vi "Initialize.vi"(8 "error in":errorcluster, 9 "Number of Channels":u32=1, 10 "Plugin Name":string, 11 "Cycler in":refnum<class "Cycler.lvclass">) -> (0 "error out":errorcluster, 3 "Cycler out":refnum<class "Cycler.lvclass">)   [LabVIEW 2023, in "Cycler.lvclass"]
doc: "This VI initializes required data channels for a Cycler. Wire the number of power output channels to <b>Number of Channels</b>, the default is 1."
uses:
  Cycler.lvclass
  Cycler.lvclass/Cycler.ctl
  <vilib>/ADAS Replay HIL/Channels/Tag Wrapper/Polymorphic/Open Producer Tag (Double).vi
  <vilib>/ADAS Replay HIL/Channels/Tag Wrapper/Polymorphic/Set Default Value (Double).vi
  <vilib>/ADAS Replay HIL/Channels/Tag Wrapper/Polymorphic/Open Consumer Tag (Boolean).vi
  <vilib>/ADAS Replay HIL/Channels/Tag Wrapper/Polymorphic/Set Default Value (Boolean).vi
  <vilib>/ADAS Replay HIL/Channels/Tag Wrapper/Polymorphic/Open Producer Tag (Boolean).vi
  <vilib>/ADAS Replay HIL/Channels/Tag Wrapper/Polymorphic/Open Producer Tag (Double).vi/45cd6eaa-a1ce-41a4-8aba-62a49d103d7e.vi
  <vilib>/ADAS Replay HIL/Channels/Tag Wrapper/Polymorphic/Set Default Value (Double).vi/228e99de-6fcf-414d-86fc-dc277c7b351f.vi
  <vilib>/ADAS Replay HIL/Channels/Tag Wrapper/Polymorphic/Open Consumer Tag (Boolean).vi/bacb721e-673a-491a-accd-959f2e1f334e.vi
  <vilib>/ADAS Replay HIL/Channels/Tag Wrapper/Polymorphic/Set Default Value (Boolean).vi/228e99de-6fcf-414d-86fc-dc277c7b351f.vi
  <vilib>/ADAS Replay HIL/Channels/Tag Wrapper/Polymorphic/Open Producer Tag (Boolean).vi/45cd6eaa-a1ce-41a4-8aba-62a49d103d7e.vi
  <vilib>/ADAS Replay HIL/Channels/Tag Wrapper/Polymorphic/Open Producer Tag (Double).vi/45cd6eaa-a1ce-41a4-8aba-62a49d103d7e.vi/c28b0ead-42ad-4072-80a2-aca7f2bd7ce3.vi
  <vilib>/ADAS Replay HIL/Channels/Tag Wrapper/Polymorphic/Set Default Value (Double).vi/228e99de-6fcf-414d-86fc-dc277c7b351f.vi/4bc1c15b-36ab-481f-b8dd-c64075ce723a.vi
  <vilib>/ADAS Replay HIL/Channels/Tag Wrapper/Polymorphic/Open Consumer Tag (Boolean).vi/bacb721e-673a-491a-accd-959f2e1f334e.vi/c28b0ead-42ad-4072-80a2-aca7f2bd7ce3.vi
  <vilib>/ADAS Replay HIL/Channels/Tag Wrapper/Polymorphic/Set Default Value (Boolean).vi/228e99de-6fcf-414d-86fc-dc277c7b351f.vi/4bc1c15b-36ab-481f-b8dd-c64075ce723a.vi
  <vilib>/ADAS Replay HIL/Channels/Tag Wrapper/Polymorphic/Open Producer Tag (Boolean).vi/45cd6eaa-a1ce-41a4-8aba-62a49d103d7e.vi/c28b0ead-42ad-4072-80a2-aca7f2bd7ce3.vi
  <vilib>/ADAS Replay HIL/AdasHilServices/AdasHilServices Fill In Error Info Ex.vi
  <vilib>/ADAS Replay HIL/Channels/Tag Wrapper/Tag Wrapper.lvlib
  Utilities/Utilities.lvlib
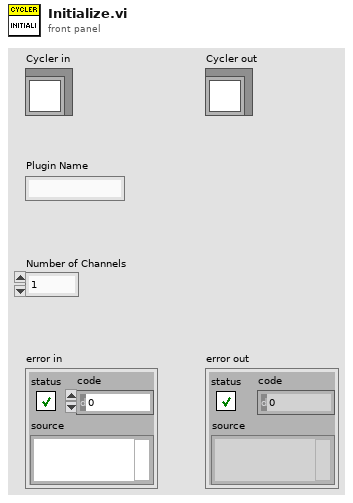
[diagram p1: front panel]
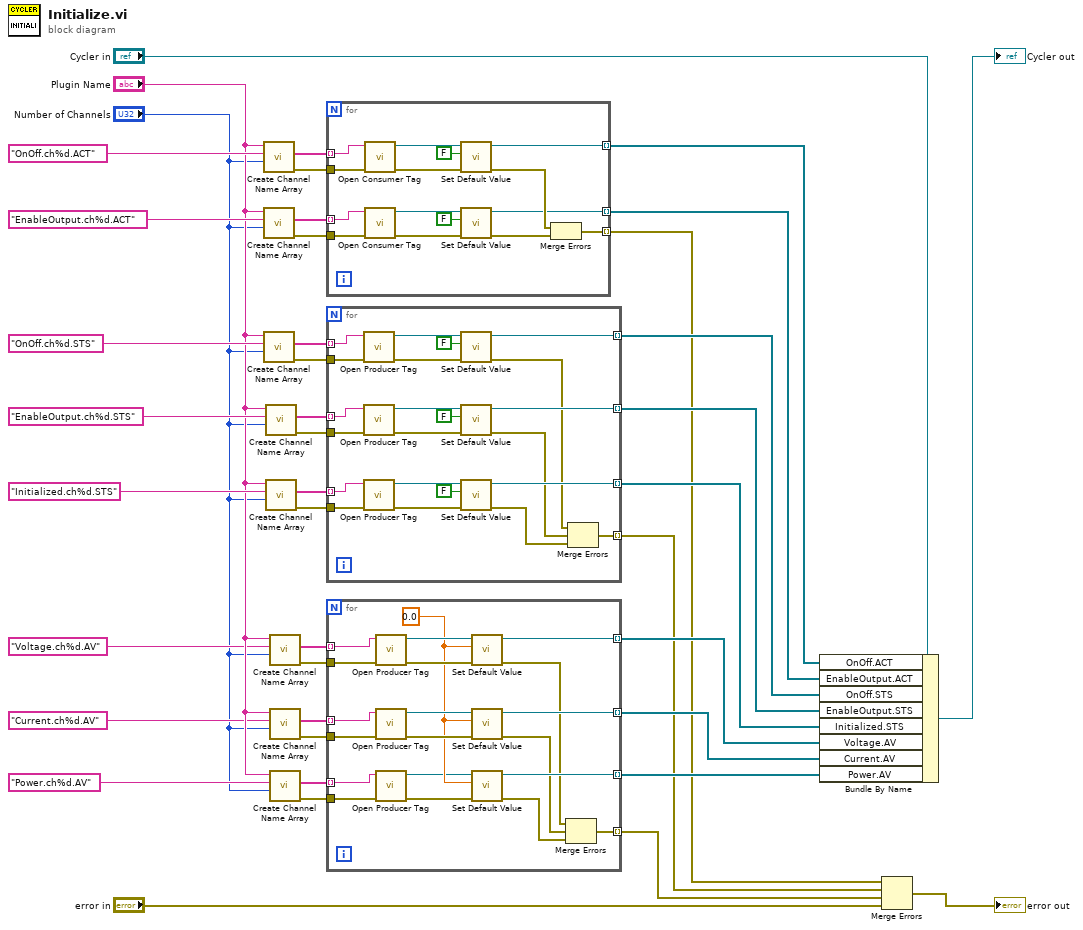
[diagram p0: block diagram]
diagram:
  n1 = call "Create Channel Name Array.vi"("Number of Channels"="Number of Channels", "Channel Format String"="OnOff.ch%d.ACT", "Plugin Name"="Plugin Name") -> ("error out"=w37:errorcluster, "Channel Names"=w40:string[])  [unwired: 7 in]
  n2 = call "Create Channel Name Array.vi"("Number of Channels"="Number of Channels", "Channel Format String"="EnableOutput.ch%d.ACT", "Plugin Name"="Plugin Name") -> ("error out"=w35:errorcluster, "Channel Names"=w34:string[])  [unwired: 7 in]
  n3 = call "Create Channel Name Array.vi"("Number of Channels"="Number of Channels", "Channel Format String"="OnOff.ch%d.STS", "Plugin Name"="Plugin Name") -> ("error out"=w32:errorcluster, "Channel Names"=w33:string[])  [unwired: 7 in]
  n4 = call "Create Channel Name Array.vi"("Number of Channels"="Number of Channels", "Channel Format String"="EnableOutput.ch%d.STS", "Plugin Name"="Plugin Name") -> ("error out"=w36:errorcluster, "Channel Names"=w39:string[])  [unwired: 7 in]
  n5 = call "Create Channel Name Array.vi"("Number of Channels"="Number of Channels", "Channel Format String"="Initialized.ch%d.STS", "Plugin Name"="Plugin Name") -> ("error out"=w27:errorcluster, "Channel Names"=w25:string[])  [unwired: 7 in]
  n6 = call "Create Channel Name Array.vi"("Number of Channels"="Number of Channels", "Channel Format String"="Voltage.ch%d.AV", "Plugin Name"="Plugin Name") -> ("error out"=w17:errorcluster, "Channel Names"=w18:string[])  [unwired: 7 in]
  n7 = call "Create Channel Name Array.vi"("Number of Channels"="Number of Channels", "Channel Format String"="Current.ch%d.AV", "Plugin Name"="Plugin Name") -> ("error out"=w15:errorcluster, "Channel Names"=w16:string[])  [unwired: 7 in]
  n8 = call "Create Channel Name Array.vi"("Number of Channels"="Number of Channels", "Channel Format String"="Power.ch%d.AV", "Plugin Name"="Plugin Name") -> ("error out"=w13:errorcluster, "Channel Names"=w14:string[])  [unwired: 7 in]
  n9 = for {
    tunnel: w40 -> [w56] mode=indexing
    tunnel: w37 -> [w55]
    tunnel: w35 -> [w54]
    tunnel: w34 -> [w53] mode=indexing
    tunnel: [w44] -> w6 mode=indexing
    tunnel: [w43] -> w5 mode=indexing
    tunnel: [w42] -> w4 mode=indexing
    n10 = call-poly <vilib>:"Open Consumer Tag.vi"("error in"=w55, "Channel Name"=w56) -> ("error out"=w51:errorcluster, "ADAS HIL Channel"=w52:refnum<k21>)  [unwired: 8 in]
    n11 = call-poly <vilib>:"Open Consumer Tag.vi"("error in"=w54, "Channel Name"=w53) -> ("error out"=w49:errorcluster, "ADAS HIL Channel"=w50:refnum<k21>)  [unwired: 8 in]
    n12 = call-poly <vilib>:"Set Default Value.vi"("error in"=w51, "Default Value"=FALSE, "ADAS HIL Channel in"=w52) -> ("error out"=w46:errorcluster, "ADAS HIL Channel out"=w43:refnum<k21>)  [unwired: 7 in]
    n13 = call-poly <vilib>:"Set Default Value.vi"("error in"=w49, "Default Value"=FALSE, "ADAS HIL Channel in"=w50) -> ("error out"=w45:errorcluster, "ADAS HIL Channel out"=w44:refnum<k21>)  [unwired: 7 in]
    n14 = Merge Errors(w46, w45) -> (w42:errorcluster)
  }
  n15 = for {
    tunnel: w39 -> [w78] mode=indexing
    tunnel: w36 -> [w77]
    tunnel: w33 -> [w76] mode=indexing
    tunnel: w32 -> [w75]
    tunnel: w27 -> [w74]
    tunnel: w25 -> [w73] mode=indexing
    tunnel: [w63] -> w7 mode=indexing
    tunnel: [w62] -> w8 mode=indexing
    tunnel: [w61] -> w9 mode=indexing
    tunnel: [w57] -> w3 mode=indexing
    n16 = call-poly <vilib>:"Open Producer Tag.vi"("error in"=w75, "Channel Name"=w76) -> ("error out"=w67:errorcluster, "ADAS HIL Channel"=w68:refnum<k21>)  [unwired: 8 in]
    n17 = call-poly <vilib>:"Open Producer Tag.vi"("error in"=w77, "Channel Name"=w78) -> ("error out"=w70:errorcluster, "ADAS HIL Channel"=w69:refnum<k21>)  [unwired: 8 in]
    n18 = call-poly <vilib>:"Open Producer Tag.vi"("error in"=w74, "Channel Name"=w73) -> ("error out"=w72:errorcluster, "ADAS HIL Channel"=w71:refnum<k21>)  [unwired: 8 in]
    n19 = call-poly <vilib>:"Set Default Value.vi"("error in"=w67, "Default Value"=FALSE, "ADAS HIL Channel in"=w68) -> ("error out"=w60:errorcluster, "ADAS HIL Channel out"=w63:refnum<k21>)  [unwired: 7 in]
    n20 = call-poly <vilib>:"Set Default Value.vi"("error in"=w70, "Default Value"=FALSE, "ADAS HIL Channel in"=w69) -> ("error out"=w59:errorcluster, "ADAS HIL Channel out"=w62:refnum<k21>)  [unwired: 7 in]
    n21 = call-poly <vilib>:"Set Default Value.vi"("error in"=w72, "Default Value"=FALSE, "ADAS HIL Channel in"=w71) -> ("error out"=w58:errorcluster, "ADAS HIL Channel out"=w61:refnum<k21>)  [unwired: 7 in]
    n22 = Merge Errors(w60, w59, w58) -> (w57:errorcluster)
  }
  n23 = for {
    tunnel: w18 -> [w98] mode=indexing
    tunnel: [w96] -> w12 mode=indexing
    tunnel: w17 -> [w95]
    tunnel: w16 -> [w93] mode=indexing
    tunnel: w15 -> [w92]
    tunnel: [w90] -> w11 mode=indexing
    tunnel: w14 -> [w86] mode=indexing
    tunnel: w13 -> [w85]
    tunnel: [w83] -> w10 mode=indexing
    tunnel: [w79] -> w2 mode=indexing
    w88 = 0.0 ("Default Value")
    n24 = call-poly <vilib>:"Open Producer Tag.vi"("error in"=w95, "Channel Name"=w98) -> ("error out"=w94:errorcluster, "ADAS HIL Channel"=w97:refnum<k21>)  [unwired: 8 in]
    n25 = call-poly <vilib>:"Open Producer Tag.vi"("error in"=w92, "Channel Name"=w93) -> ("error out"=w89:errorcluster, "ADAS HIL Channel"=w91:refnum<k21>)  [unwired: 8 in]
    n26 = call-poly <vilib>:"Open Producer Tag.vi"("error in"=w85, "Channel Name"=w86) -> ("error out"=w84:errorcluster, "ADAS HIL Channel"=w87:refnum<k21>)  [unwired: 8 in]
    n27 = call-poly <vilib>:"Set Default Value.vi"("error in"=w94, "Default Value"=w88, "ADAS HIL Channel in"=w97) -> ("error out"=w82:errorcluster, "ADAS HIL Channel out"=w96:refnum<k21>)  [unwired: 7 in]
    n28 = call-poly <vilib>:"Set Default Value.vi"("error in"=w89, "Default Value"=w88, "ADAS HIL Channel in"=w91) -> ("error out"=w81:errorcluster, "ADAS HIL Channel out"=w90:refnum<k21>)  [unwired: 7 in]
    n29 = call-poly <vilib>:"Set Default Value.vi"("error in"=w84, "Default Value"=w88, "ADAS HIL Channel in"=w87) -> ("error out"=w80:errorcluster, "ADAS HIL Channel out"=w83:refnum<k21>)  [unwired: 7 in]
    n30 = Merge Errors(w82, w81, w80) -> (w79:errorcluster)
  }
  n31 = Bundle By Name(cluster="Cycler in", "OnOff.ACT"=w5, "EnableOutput.ACT"=w6, "OnOff.STS"=w7, "EnableOutput.STS"=w8, "Initialized.STS"=w9, "Voltage.AV"=w12, "Current.AV"=w11, "Power.AV"=w10) -> (→"Cycler out":refnum<class "Cycler.lvclass">)
  n32 = Merge Errors(w4, w3, w2, "error in") -> (→"error out":errorcluster)
